vi "The ChapR.vi"(9 "Position":u8=49, 10 "Alliance":u8=66, 11 "TeamNo (4 digits)":u16=2468) -> ()   [LabVIEW 2013]
doc: "*Does NOT need to be changed*\n\nInputs:\nTeamNo (optional; default - 2468)\nAlliance (optional; default - 66)\nPosition (optional; default - 49)\n\nDescription:\nA VI to take in input over Bluetooth from the ChapR, and designed to be used with a Bluetooth to Serial converter plugged into the cRIO. It takes the serial data, decomposes it into ChapR packets, then translates those into FMS packets and sends them to itself (so the TeleOp portions of Main.vi respond appropriately)."
uses:
  ChapR Packet.ctl
  <vilib>/Instr/_visa.llb/VISA Configure Serial Port (Instr).vi
panel:
  out "bad packets":T1
  in  "connection ID":refnum<k16>
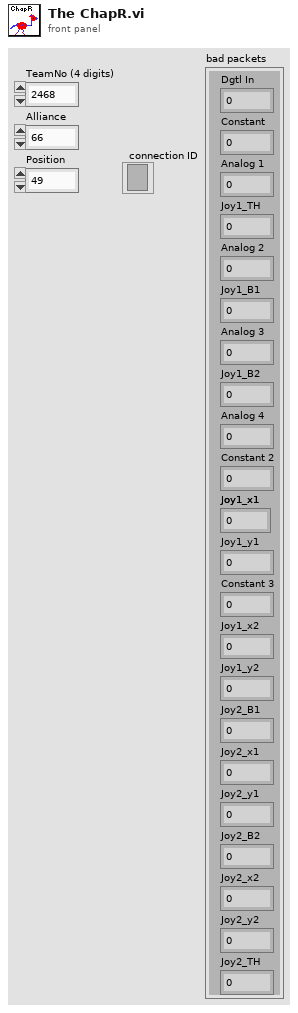
[diagram p1: front panel]
types:
  T1 = typedef "ChapR Packet.ctl" = cluster{"Dgtl In":u8, "Constant":u8, "Analog 1":u16, "Joy1_TH":u8, "Analog 2":u16, "Joy1_B1":u8, "Analog 3":u16, "Joy1_B2":u8, "Analog 4":u16, "Constant 2":u8, "Joy1_x1":i8, "Joy1_y1":i8, "Constant 3":u8, "Joy1_x2":i8, "Joy1_y2":i8, "Joy2_B1":u8, "Joy2_x1":i8, "Joy2_y1":i8, "Joy2_B2":u8, "Joy2_x2":i8, "Joy2_y2":i8, "Joy2_TH":u8}
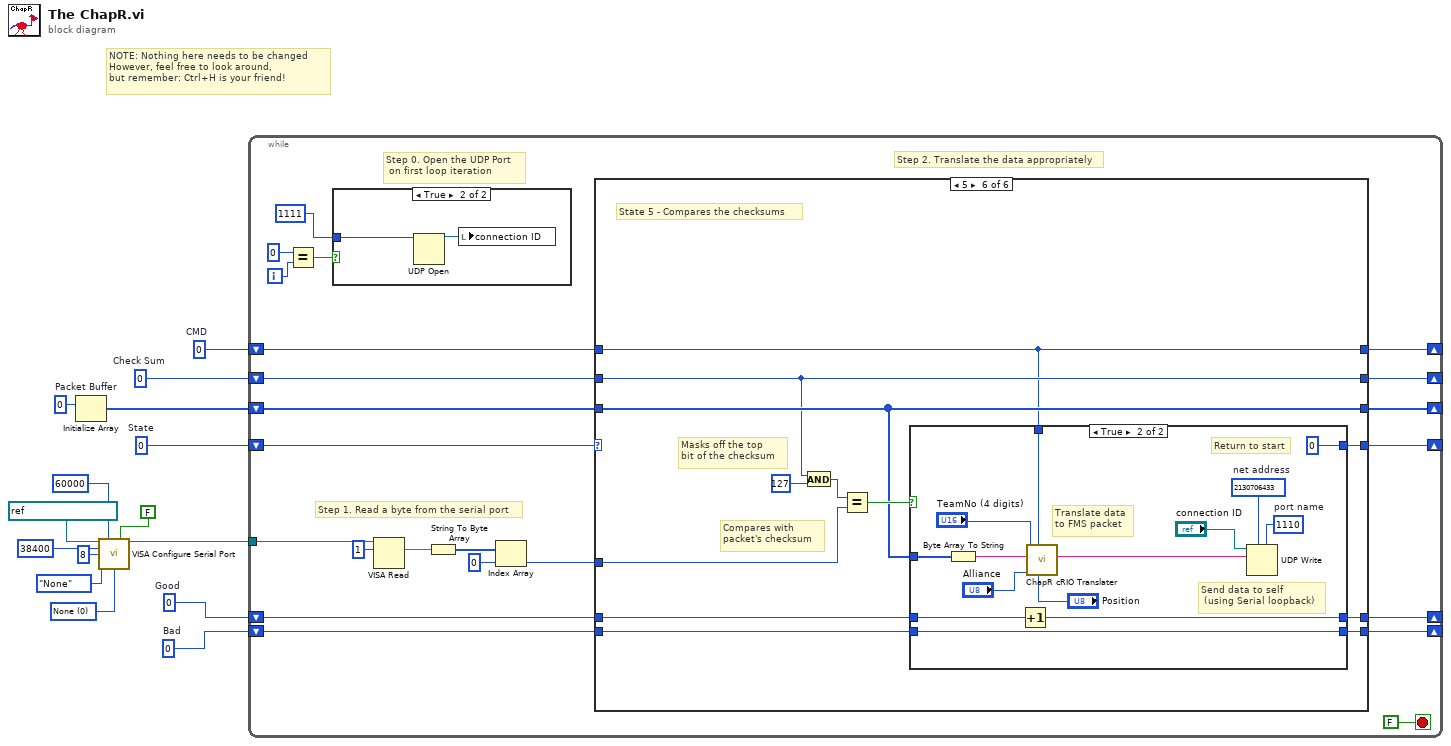
[diagram p0: block diagram]
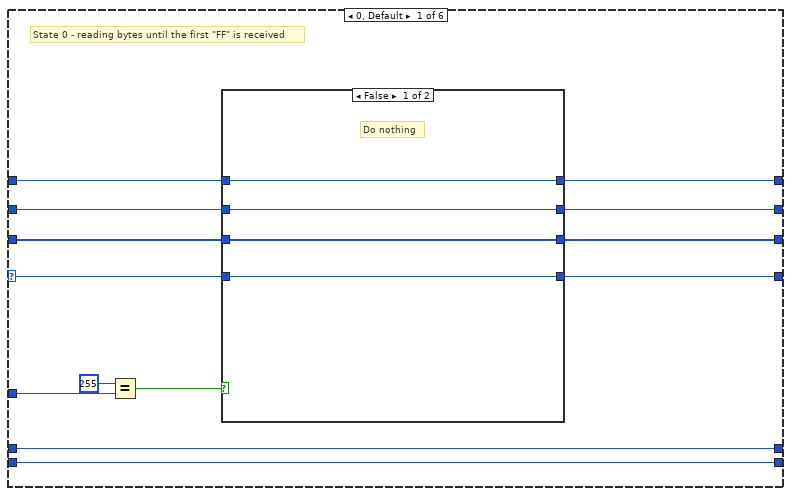
[diagram p3: hidden frame]
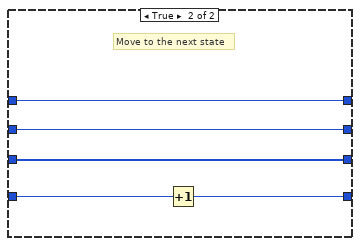
[diagram p4: hidden frame]
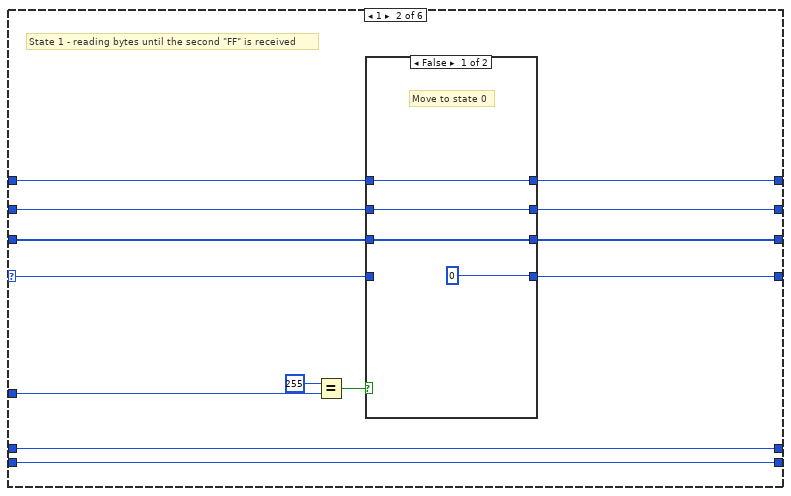
[diagram p5: hidden frame]
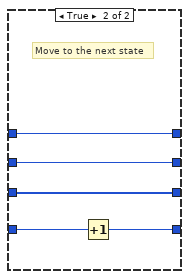
[diagram p6: hidden frame]
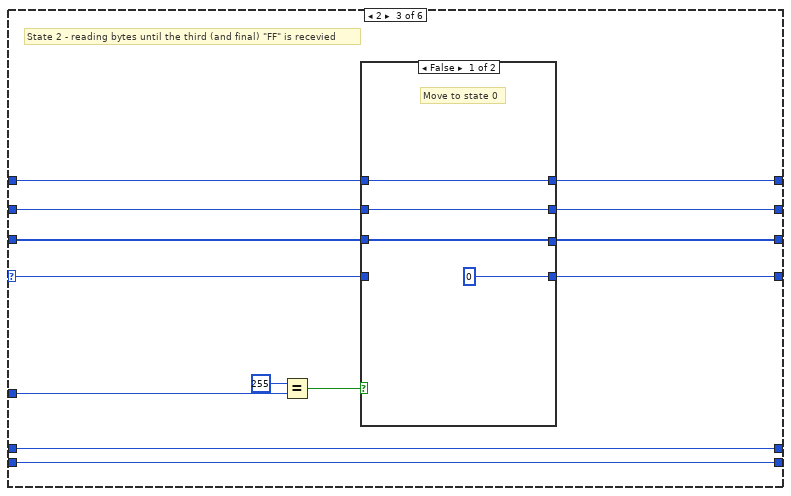
[diagram p7: hidden frame]
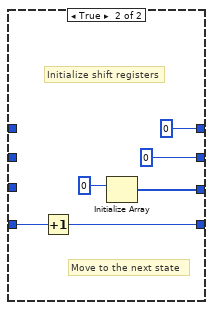
[diagram p8: hidden frame]
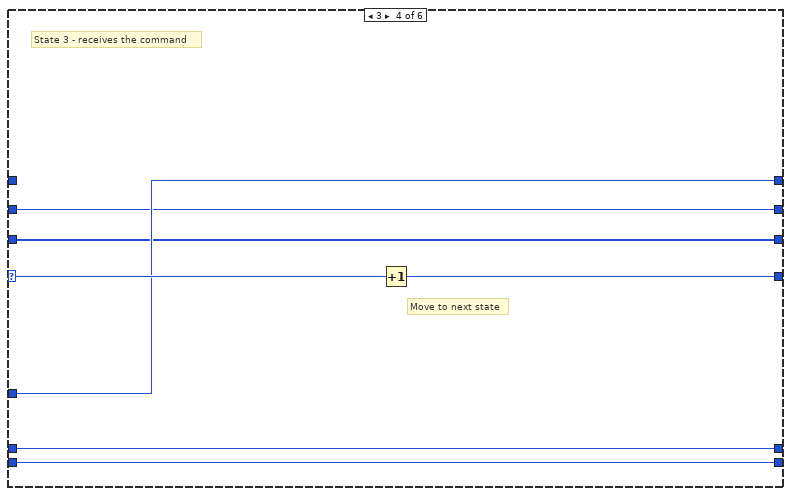
[diagram p9: hidden frame]
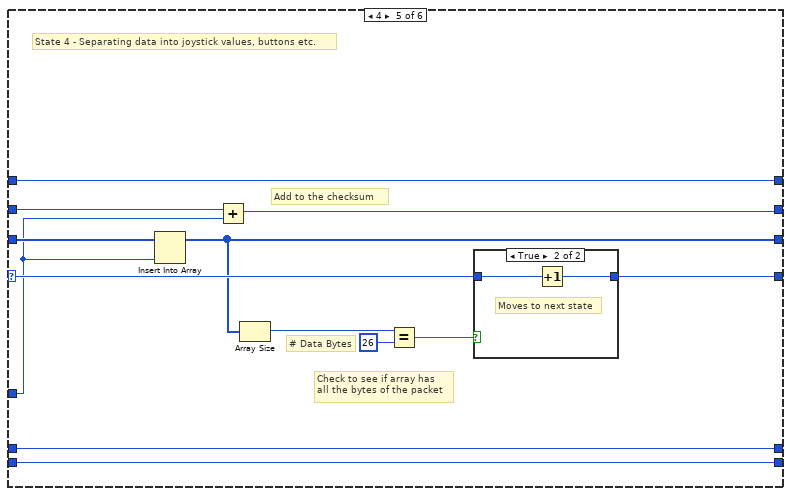
[diagram p10: hidden frame]
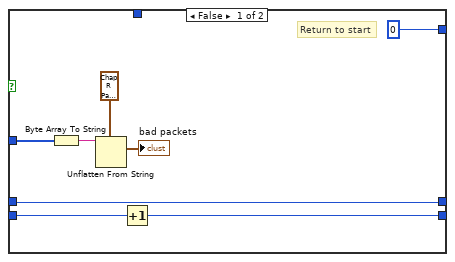
[diagram p12: hidden frame]
diagram:
  w1 = u16 0 items=["None", "XON/XOFF", "RTS/CTS", "XON/XOFF & RTS/CTS", "DTR/DSR", "XON/XOFF & DTR/DSR"] ("flow control (0:none)")
  w11 = 0  # Bad
  w12 = 0  # Good
  w9 = u8 0  # CMD
  w10 = u8 0  # Check Sum
  w15 = 0  # State
  # "NOTE: Nothing here needs to be changed\nHowever, feel free to look around, \nbut remember: Ctrl+H is your friend!"
  n1 = Initialize Array "Packet Buffer"(u8 0 ("element")) -> (w14:u8[])  [unwired: 1 in]
  n2 = call-poly "VISA Configure Serial Port"("VISA resource name"=refnum<visa-resource-name> "ASRL1::INSTR", "timeout (10sec)"=u32 60000, "Enable Termination\nChar (T)"=FALSE ("Enable Termination\nChar (T)"), "baud rate (9600)"=u32 38400, "data bits (8)"=u16 8, "parity (0:none)"=enum16{"None", "Odd", "Even", "Mark", "Space"}."None", "flow control (0:none)"=w1) -> ("VISA resource name out"=w2:refnum<visa-resource-name>)  [unwired: 7 in, 1 out]
  n3 = while {
    shift-right: [w36] -> _
    shift-left: w15 -> [w37]
    shift-right: [w28] -> _
    shift-left: w10 -> [w29]
    shift-right: [w34] -> _
    shift-left: w14 -> [w35]
    shift-right: [w30] -> _
    shift-left: w12 -> [w33]
    shift-right: [w31] -> _
    shift-left: w11 -> [w32]
    shift-right: [w26] -> _
    shift-left: w9 -> [w27]
    tunnel: w2 -> [w17]
    i -> [w24]
    stop <- FALSE stop-if-true
    # "Step 0. Open the UDP Port\n on first loop iteration"
    # "Step 2. Translate the data appropriately"
    # "Step 1. Read a byte from the serial port"
    n4 = Equal?(x=0, y=w24) -> (x = y?=w25:bool)
    n5 = case shown="True" w25 {
      tunnel: u16 1111 ("port") -> [_ w39]
      frame False {
      }
      frame True {
        n6 = UDP Open(11:w39) -> (port=w40:refnum<k16>)  [unwired: 4 in, 2 out]
        n7 = local write "connection ID"(w40) -> ()
      }
    }
    n8 = VISA Read(VISA resource name=w17, byte count=u32 1) -> (read buffer=w19:string)  [unwired: 1 in, 3 out]
    n9 = String To Byte Array(string=w19) -> (unsigned byte array=w20:u8[])
    n10 = Index Array(array=w20, index=0) -> (element=w16:u8)
    n11 = case shown="5" w37 {
      selector: w37 -> [w52 w74 w97 w114 w126 _]
      tunnel: [w51 w73 w96 w113 w127 w141] -> w36
      tunnel: [w45 w65 w87 w108 w124 w132] -> w28
      tunnel: [w43 w63 w85 w112 w116 w131] -> w26
      tunnel: w16 -> [w49 w71 w93 w112 w122 w138]
      tunnel: w35 -> [w48 w70 w91 w111 w123 w137]
      tunnel: [w47 w69 w92 w111 w115 w137] -> w34
      tunnel: w33 -> [w42 w68 w90 w110 w119 w134]
      tunnel: w32 -> [w41 w67 w89 w109 w118 w136]
      tunnel: [w41 w67 w89 w109 w118 w135] -> w31
      tunnel: [w42 w68 w90 w110 w119 w133] -> w30
      tunnel: w29 -> [w46 w66 w88 w108 w117 w132]
      tunnel: w27 -> [w44 w64 w86 _ w116 w131]
      frame 0, Default {
        # "State 0 - reading bytes until the first \"FF\" is received"
        n12 = Equal?(x=u8 255, y=w49) -> (x = y?=w53:bool)
        n13 = case shown="False" w53 {
          tunnel: w52 -> [w57 w62]
          tunnel: [w57 w61] -> w51
          tunnel: w48 -> [w56 w60]
          tunnel: [w56 w60] -> w47
          tunnel: [w55 w59] -> w45
          tunnel: w46 -> [w55 w59]
          tunnel: [w54 w58] -> w43
          tunnel: w44 -> [w54 w58]
          frame False {
            # "Do nothing"
          }
          frame True {
            # "Move to the next state"
            n14 = Increment(x=w62) -> (x+1=w61:i32)
          }
        }
      }
      frame 1 {
        # "State 1 - reading bytes until the second \"FF\" is received"
        n15 = Equal?(x=u8 255, y=w71) -> (x = y?=w75:bool)
        n16 = case shown="False" w75 {
          tunnel: w74 -> [_ w84]
          tunnel: [0 w83] -> w73
          tunnel: w70 -> [w79 w82]
          tunnel: [w79 w82] -> w69
          tunnel: [w78 w81] -> w65
          tunnel: w66 -> [w78 w81]
          tunnel: [w77 w80] -> w63
          tunnel: w64 -> [w77 w80]
          frame False {
            # "Move to state 0"
          }
          frame True {
            # "Move to the next state"
            n17 = Increment(x=w84) -> (x+1=w83:i32)
          }
        }
      }
      frame 2 {
        # "State 2 - reading bytes until the third (and final) \"FF\" is recevied"
        n18 = Equal?(x=u8 255, y=w93) -> (x = y?=w94:bool)
        n19 = case shown="False" w94 {
          tunnel: [0 w106] -> w96
          tunnel: w97 -> [_ w107]
          tunnel: [w100 u8 0] -> w87
          tunnel: [w99 u8 0] -> w85
          tunnel: [w101 w102] -> w92
          tunnel: w91 -> [w101 _]
          tunnel: w88 -> [w100 _]
          tunnel: w86 -> [w99 _]
          frame False {
            # "Move to state 0"
          }
          frame True {
            # "Initialize shift registers"
            # "Move to the next state"
            n20 = Increment(x=w107) -> (x+1=w106:i32)
            n21 = Initialize Array ("Packet Buffer")(u8 0 ("element")) -> (w102:u8[])  [unwired: 1 in]
          }
        }
      }
      frame 3 {
        # "Move to next state"
        # "State 3 - receives the command"
        n22 = Increment(x=w114) -> (x+1=w113:i32)
      }
      frame 4 {
        # "Check to see if array has \nall the bytes of the packet"
        # "Add to the checksum"
        # "# Data Bytes"
        # "State 4 - Separating data into joystick values, buttons etc."
        n23 = Insert Into Array(array=w123, new element=w122) -> (w115:u8[])  [unwired: 1 in]
        n24 = Add(x=w117, y=w122) -> (x+y=w124:u8)
        n25 = Array Size(array=w115) -> (size(s)=w121:i32)
        n26 = Equal?(x=w121, y=26) -> (x = y?=w120:bool)
        n27 = case shown="True" w120 {
          tunnel: [w128 w129] -> w127
          tunnel: w126 -> [w128 w130]
          frame False {
            # "Do nothing"
          }
          frame True {
            # "Moves to next state"
            n28 = Increment(x=w130) -> (x+1=w129:i32)
          }
        }
      }
      frame 5 {
        # "Compares with \npacket's checksum"
        # "Masks off the top \nbit of the checksum"
        # "State 5 - Compares the checksums"
        n29 = And(x=w132, y=u8 127) -> (x .and. y?=w140:u8)
        n30 = Equal?(x=w140, y=w138) -> (x = y?=w142:bool)
        n31 = case shown="True" w142 {
          tunnel: [0 0] -> w141
          tunnel: w137 -> [w148 w163]
          tunnel: w136 -> [w146 w162]
          tunnel: [w145 w162] -> w135
          tunnel: w134 -> [w144 w161]
          tunnel: [w144 w160] -> w133
          tunnel: w131 -> [_ w151]
          frame False {
            # "Return to start"
            n32 = Byte Array To String(unsigned byte array=w148) -> (string=w147:string)
            n33 = Unflatten From String(type=T1 {"Dgtl In"=0, "Constant"=0, "Analog 1"=0, "Joy1_TH"=0, "Analog 2"=0, "Joy1_B1"=0, "Analog 3"=0, "Joy1_B2"=0, "Analog 4"=0, "Constant 2"=0, "Joy1_x1"=0, "Joy1_y1"=0, "Constant 3"=0, "Joy1_x2"=0, "Joy1_y2"=0, "Joy2_B1"=0, "Joy2_x1"=0, "Joy2_y1"=0, "Joy2_B2"=0, "Joy2_x2"=0, "Joy2_y2"=0, "Joy2_TH"=0}, binary string=w147) -> (value=→"bad packets":T1)  [unwired: 3 in, 2 out]
            n34 = Increment(x=w146) -> (x+1=w145:i32)
          }
          frame True {
            w152 = u16 1110  # port name
            w155 = u32 2130706433  # net address
            # "Return to start"
            # "Send data to self\n (using Serial loopback)"
            # "Translate data \nto FMS packet"
            n35 = Byte Array To String(unsigned byte array=w163) -> (string=w159:string)
            n36 = Increment(x=w161) -> (x+1=w160:i32)
            n37 = call "ChapR cRIO Translater.vi"("Position"="Position", "CMD"=w151, "Alliance"="Alliance", "ChapR Data"=w159, "TeamNo"="TeamNo (4 digits)") -> ("Network Data"=w154:string)  [unwired: 6 in]
            n38 = UDP Write(address=w155, port or service name=w152, connection ID="connection ID", data in=w154) -> ()  [unwired: 2 in, 2 out]
          }
        }
      }
    }
  }
